vi "Preview_Worksheet.vi"(8 "error in (no error)":errorcluster, 10 "Path":path, 11 "ExcelFile in":refnum<class "PortableExcelFileManipulationOXML.lvclass">) -> (0 "error out":errorcluster, 2 "Report Path":path, 3 "ExcelFile out":refnum<class "PortableExcelFileManipulationOXML.lvclass">)   [LabVIEW 2019, in "PortableExcelFileManipulationOXML.lvclass"]
doc: "Converts document to PDF inside temporary directory, then opens pdf with default application."
uses:
  PortableExcelFileManipulationOXML.lvclass
  PortableExcelFileManipulationOXML.lvclass/PortableExcelFileManipulationOXML.ctl
  H:/LV projects/ExpressionEvaluator/Excel/ExcelManipulation.dll
  ExcelManipulation.dll
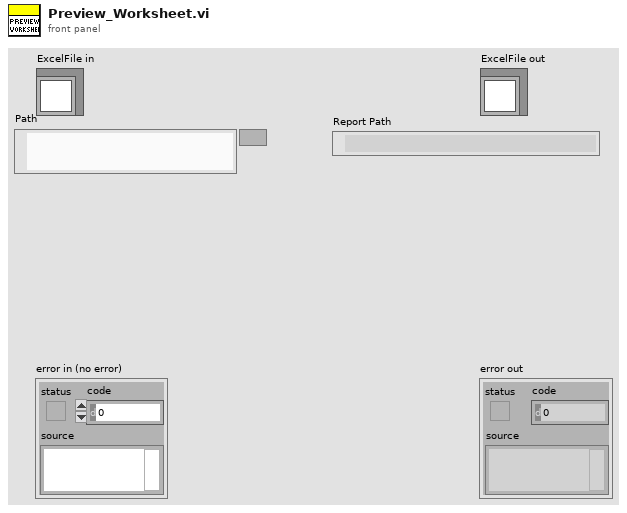
[diagram p1: front panel]
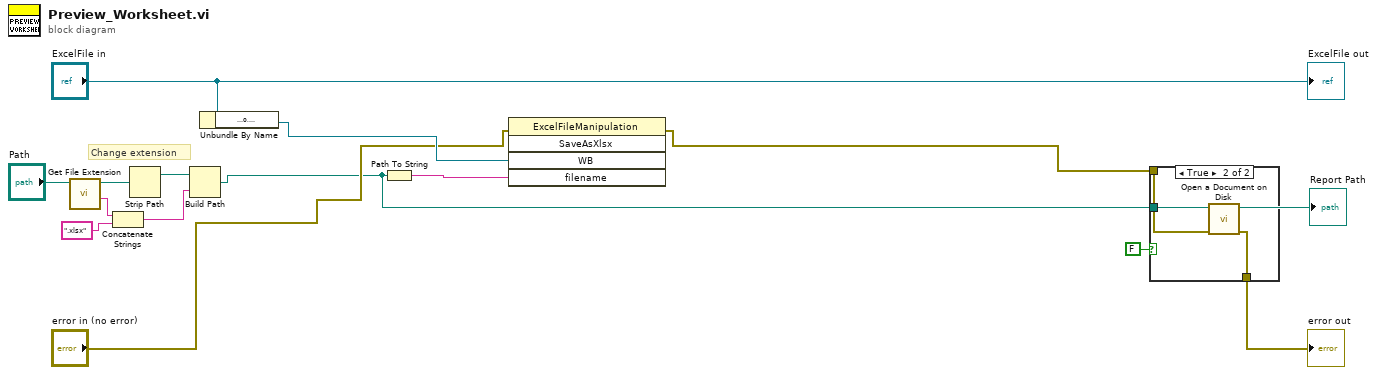
[diagram p0: block diagram]
diagram:
  # "Change extension"
  n1 = call <vilib>:"Get File Extension.vi"("file"="Path") -> ("filename without extension"=w7:string, "dup file"=w5:path)  [unwired: 6 in, 3 out]
  n2 = Concatenate Strings(w7, ".xlsx" ("string")) -> (w8:string)
  n3 = Strip Path(path=w5) -> (stripped path=w6:path)  [unwired: 1 out]
  n4 = Build Path(base path=w6, name or relative path=w8) -> (appended path=w3:path)
  "Report Path" <- w3
  n5 = Unbundle By Name("ExcelFile in") -> ("ExcelOpen"=w11:refnum<k24>)
  n6 = Path To String(path=w3) -> (string=w10:string)
  n7 = invoke class="ExcelFileManipulation" method="SaveAsXlsx"(error in="error in (no error)", "WB"=w11, "filename"=w10) -> (error out=w9:errorcluster)  [unwired: 2 in, 4 out]
  n8 = case shown="True" FALSE {
    tunnel: [w15 w18] -> w14
    tunnel: w3 -> [_ w17]
    tunnel: w9 -> [w15 w16]
    frame False {
    }
    frame True {
      n9 = call <vilib>:"Open a Document on Disk.vi"("error in (no error)"=w16, "document path"=w17) -> ("error out"=w18:errorcluster)  [unwired: 5 in]
    }
  }
  "error out" <- w14
  "ExcelFile out" <- "ExcelFile in"
